vi "Register for gRPC Server Events.vi"(8 "error in (no error)":errorcluster, 11 "CIFLauncher in":refnum<class "CIFPluginLoader.lvclass">) -> (0 "error out":errorcluster, 1 "Discovery Event Registration Refnum":refnum<event-registration>, 2 "Main Event Registration Refnum":refnum<event-registration>, 3 "CIFLauncher out":refnum<class "CIFPluginLoader.lvclass">)   [LabVIEW 2021, in "CIFPluginLoader.lvclass"]
uses:
  CIFPluginLoader.lvclass
  CIF_PluginLoader_server/RPC Service/PluginLoader/PluginLoader.lvclass
  C:/Program Files/National Instruments/LabVIEW 2021/vi.lib/gRPC/LabVIEW gRPC Servicer/ServiceBase/ServiceBase.lvclass
  CIFPluginLoader.lvclass/CIFPluginLoader.ctl
  CIF_PluginLoader_server/RPC Service/PluginLoader/PluginLoader.lvclass/PluginLoader.ctl
  D:/dev/CIF-LVCore/src/CIFPluginManager/CIFPluginLoader/gRPC/CIF_PluginLoader_server/RPC Service/PluginLoader/PluginLoader.lvclass
  <vilib>/gRPC/LabVIEW gRPC Library/Shared/grpcId.ctl
  <vilib>/gRPC/LabVIEW gRPC Library/grpc-lvsupport-release.lvlib
  <vilib>/gRPC/LabVIEW gRPC Library/Server API/typeDefs/gRPCId Cluster.ctl
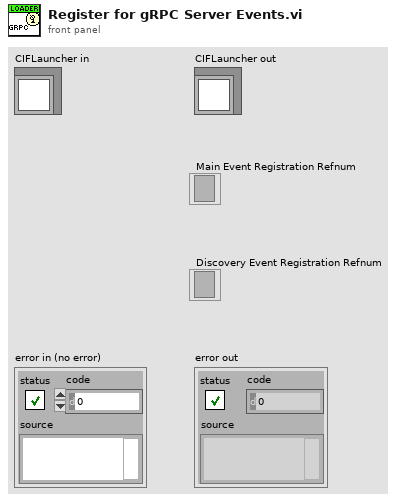
[diagram p1: front panel]
types:
  T1 = typedef "CIF_PluginLoader_server.lvlib/PluginLoader.lvclass/Server gRPC UEs.ctl" = cluster{"PluginLoader LoadPlugin gRPC UE":refnum<user-event>, "PluginLoader AbortPlugin gRPC UE":refnum<user-event>, "PluginLoader Destroy gRPC UE":refnum<user-event>, "PluginLoader Ping gRPC UE":refnum<user-event>, "PluginLoader Discover gRPC UE":refnum<user-event>}
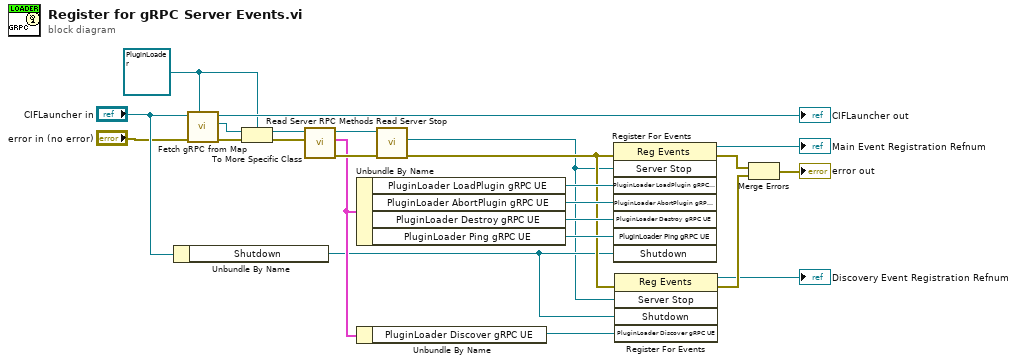
[diagram p0: block diagram]
diagram:
  w17 = refnum<class "PluginLoader.lvclass"> refnum ("CIF_PluginLoader_server.lvlib:PluginLoader.lvclass")
  n1 = Unbundle By Name("CIFLauncher in") -> ("Shutdown"=w7:refnum<user-event>)
  n2 = call "Fetch gRPC from Map.vi"("gRPC Server Class type"=w17, "error in (no error)"="error in (no error)", "CIFLauncher in"="CIFLauncher in") -> ("error out"=w15:errorcluster, "gRPC Server Class out"=w16:refnum<class "ServiceBase.lvclass">, "CIFLauncher out"=→"CIFLauncher out":refnum<class "CIFPluginLoader.lvclass">)  [unwired: 6 in]
  n3 = To More Specific Class(target class=w17, reference=w16, error in=w15) -> (specific class reference=w23:refnum<class "PluginLoader.lvclass">, error out=w21:errorcluster)
  n4 = call "Read Server RPC Methods.vi"("error in (no error)"=w21, "gRPC service in"=w23) -> ("error out"=w22:errorcluster, "Server RPC Methods"=w9:T1, "gRPC service out"=w24:refnum<class "PluginLoader.lvclass">)  [unwired: 7 in]
  n5 = Unbundle By Name(w9) -> ("PluginLoader LoadPlugin gRPC UE"=w14:refnum<user-event>, "PluginLoader AbortPlugin gRPC UE"=w11:refnum<user-event>, "PluginLoader Destroy gRPC UE"=w12:refnum<user-event>, "PluginLoader Ping gRPC UE"=w13:refnum<user-event>)
  n6 = Unbundle By Name(w9) -> ("PluginLoader Discover gRPC UE"=w5:refnum<user-event>)
  n7 = call-dynamic "Read Server Stop.vi"("error in"=w22, "gRPC service in"=w24) -> ("error out"=w8:errorcluster, "Server Stop"=w6:refnum<user-event>)  [unwired: 7 in, 1 out]
  n8 = register-events(error in=w8, w6, w14, w11, w12, w13, w7) -> (reference out=→"Main Event Registration Refnum":refnum<event-registration>, error out=w3:errorcluster)  [unwired: 1 in]
  n9 = register-events(error in=w8, w6, w7, w5) -> (reference out=→"Discovery Event Registration Refnum":refnum<event-registration>, error out=w4:errorcluster)  [unwired: 1 in]
  n10 = Merge Errors(w3, w4) -> (→"error out":errorcluster)
